vi "TeilB.vi"() -> ()   [LabVIEW 2010]
panel:
  in  "Temp Step":dbl=0.1 format="%.2f"
  in  "Temp Stop":dbl=205.0 format="%.2f"
  in  "Temp Start":dbl format="%.2f"
  in  "address Freq":string="19"
  out "Frequenz in Hz":dbl=200.0 format="%.2f"
  in  "Wait/s":dbl=1.0 format="%.2f"
  in  "Freq Step":dbl=1.0 format="%.2f"
  out "current frequency value":string
  out "error out 2":errorcluster
  in  "error in (no error) 2":errorcluster
  in  "Freq Stop":dbl=205.0 format="%.2f"
  in  "Freq Start":dbl=200.0 format="%.2f"
  in  "address LockIn":string="7"
  in  "Path":path=path "/home/fpuser1567/Downloads/Teil B/test"
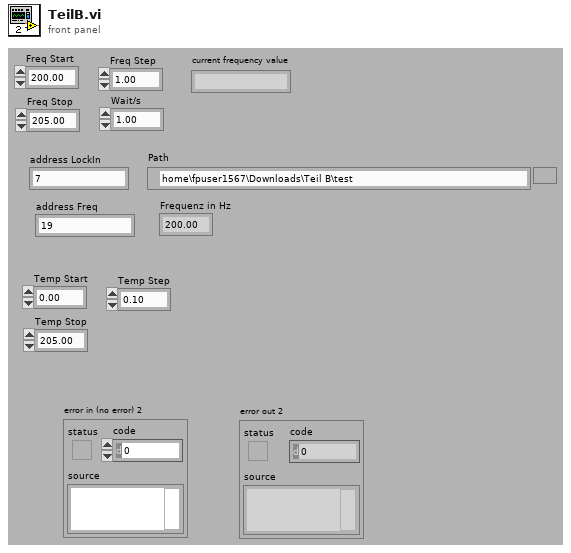
[diagram p1: front panel]
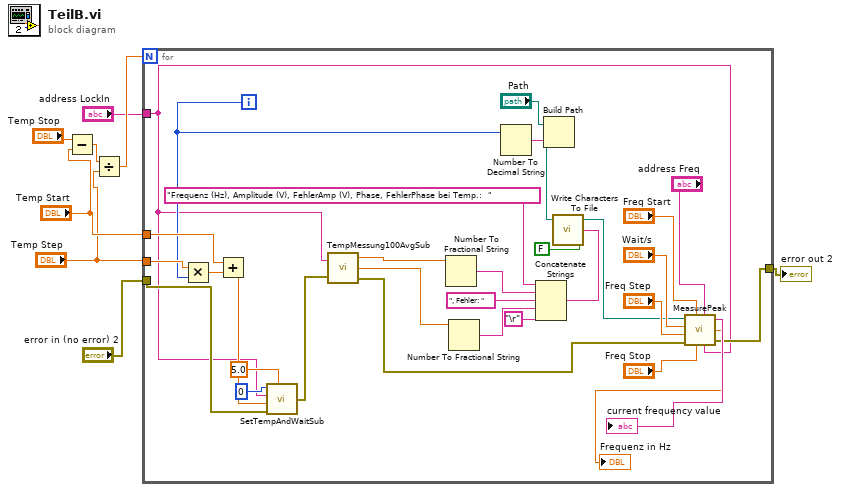
[diagram p0: block diagram]
diagram:
  n1 = Subtract(x="Temp Stop", y="Temp Start") -> (x-y=w7:dbl)
  n2 = Divide(x=w7, y="Temp Step") -> (x/y=w6:dbl)
  n3 = for {
    N: w6 -> [_]
    tunnel: "Temp Start" -> [w32]
    tunnel: "Temp Step" -> [w30]
    tunnel: "error in (no error) 2" -> [w19]
    tunnel: [w25] -> w2
    tunnel: "address LockIn" -> [w15]
    i -> [w26]
    n4 = Multiply(x=w30, y=w26) -> (x*y=w31:dbl)
    n5 = Add(x=w32, y=w31) -> (x+y=w18:dbl)
    n6 = call "SetTempAndWaitSub.vi"("mode (0)"=i16 0, "address string"=w15, "Heizspannung (V)"=w18, "error in"=w19, "Wartezeit zw. Temperaturmessungen"=5.0) -> ("error out"=w16:errorcluster)
    n7 = call "TempMessung100AvgSub.vi"("error out"=w16, "address LockIn"=w15) -> ("error out 2"=w17:errorcluster, "Numeric"=w12:dbl, "mean"=w14:dbl)
    n8 = Number To Fractional String(number=w14) -> (F-format string=w13:string)  [unwired: 3 in]
    n9 = Number To Fractional String(number=w12) -> (F-format string=w10:string)  [unwired: 3 in]
    n10 = Number To Decimal String(number=w26) -> (decimal integer string=w24:string)  [unwired: 1 in]
    n11 = Concatenate Strings("Frequenz (Hz), Amplitude (V), FehlerAmp (V), Phase, FehlerPhase bei Temp.:  ", w13, ", Fehler: ", w10, "\r") -> (w37:string)
    n12 = Build Path(base path="Path", name or relative path=w24) -> (appended path=w23:path)
    n13 = call <vilib>:"Write Characters To File.vi"("append to file? (new file:F)"=FALSE, "character string"=w37, "file path (dialog if empty)"=w23) -> ("new file path (Not A Path if cancelled)"=w22:path)  [unwired: 2 in]
    n14 = call "MeasurePeak.vi"("address Freq"="address Freq", "address LockIn"=w15, "Freq Start"="Freq Start", "Path"=w22, "Wait/s"="Wait/s", "Stop"="Freq Stop", "Step"="Freq Step", "error in (no error) 2"=w17) -> ("String"=→"current frequency value":string, "Numeric"=→"Frequenz in Hz":dbl, "error out"=w25:errorcluster)
  }
  "error out 2" <- w2
